vi "goalieLimitsInY.vi"(8 "error in (no error)":errorcluster, 9 "Goal Width/2":dbl, 10 "calculated Y":dbl format="%#_13g", 11 "DefendGoalTactic in":refnum<class "DefendGoalTactic.lvclass">) -> (0 "error out":errorcluster, 2 "coerced Y":dbl, 3 "DefendGoalTactic out":refnum<class "DefendGoalTactic.lvclass">)   [LabVIEW 2024, in "DefendGoalTactic.lvclass"]
uses:
  DefendGoalTactic.lvclass
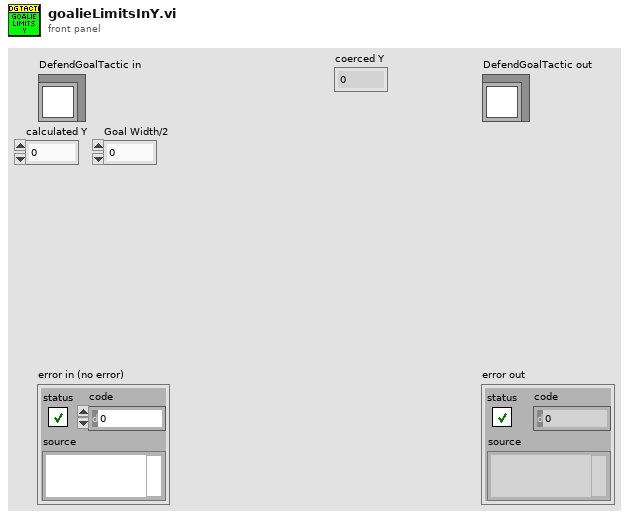
[diagram p1: front panel]
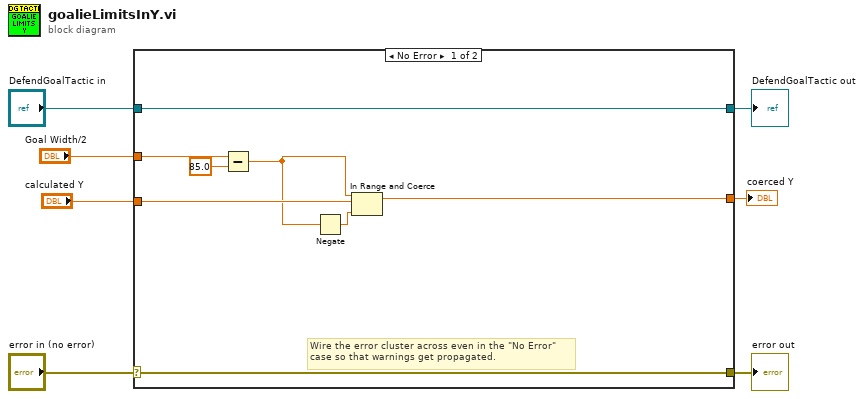
[diagram p0: block diagram]
diagram:
  n1 = case shown="No Error" "error in (no error)" {
    selector: "error in (no error)" -> [w14 w17]
    tunnel: [w14 w17] -> w6
    tunnel: [w15 w16] -> w4
    tunnel: "DefendGoalTactic in" -> [w15 w16]
    tunnel: "calculated Y" -> [w13 _]
    tunnel: "Goal Width/2" -> [w10 _]
    tunnel: [w11 _] -> w1
    frame No Error {
      # "Wire the error cluster across even in the \"No Error\"\ncase so that warnings get propagated."
      n2 = Subtract(x=w10, y=85.0) -> (x-y=w9:dbl)
      n3 = Negate(x=w9) -> (-x=w12:dbl)
      n4 = In Range and Coerce(upper limit=w9, x=w13, lower limit=w12) -> (coerced(x)=w11:dbl)  [unwired: 1 out]
    }
    frame Error {
    }
  }
  "error out" <- w6
  "DefendGoalTactic out" <- w4
  "coerced Y" <- w1
